vi "TestOpticalShutter.vi"() -> ()   [LabVIEW 2018]
uses:
  Mode.ctl
  Thorlabs_SC10.lvlib
panel:
  in  "stop":bool
  out "Toggle Shutter":bool
  in  "Mode":T1
  out "error out":errorcluster
  out "Connected?":bool
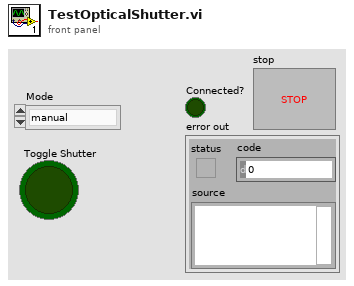
[diagram p1: front panel]
types:
  T1 = typedef "Thorlabs_SC10.lvlib/Mode.ctl" = enum16{"manual", "auto", "single", "repeat", "external gate"}
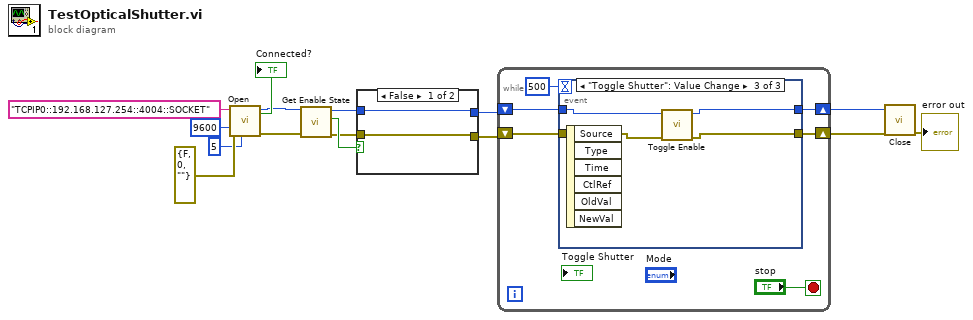
[diagram p0: block diagram]
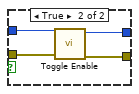
[diagram p2: hidden frame]
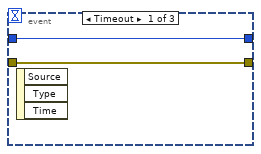
[diagram p3: hidden frame]
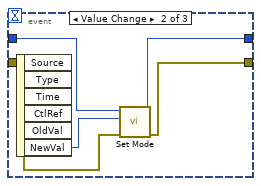
[diagram p4: hidden frame]
diagram:
  n1 = call "Open.vi"("timeout"=5, "error in (no error)"=errorcluster {"status"=FALSE, "code"=0, "source"=""}, "nbaud"=9600, "Serial Port"="TCPIP0::192.168.127.254::4004::SOCKET") -> ("error out"=w7:errorcluster, "hDevice"=w6:i32, "Connected?"=→"Connected?":bool)  [unwired: 5 in]
  n2 = call "Get Enable State.vi"("error in (no error)"=w7, "hdl"=w6) -> ("error out"=w4:errorcluster, "Enable"=w5:bool, "hdl out"=w3:i32)  [unwired: 7 in]
  n3 = case shown="False" w5 {
    tunnel: w4 -> [w16 w21]
    tunnel: w3 -> [w17 w20]
    tunnel: [w17 w19] -> w2
    tunnel: [w16 w18] -> w1
    frame False {
    }
    frame True {
      n4 = call "Toggle Enable.vi"("error in (no error)"=w21, "hdl"=w20) -> ("error out"=w18:errorcluster, "hdl out"=w19:i32)  [unwired: 8 in]
    }
  }
  n5 = while {
    shift-right: [w25] -> w9
    shift-left: w1 -> [w26]
    shift-right: [w23] -> w10
    shift-left: w2 -> [w24]
    stop <- "stop" stop-if-true
    n6 = event shown="[2] \"Toggle Shutter\": Value Change" {
      selector: _ -> [_ _ _]
      dyn-events: _ -> [_ _ _]
      timeout: 500 -> [_ _ _]
      tunnel: w26 -> [w29 w32 w37]
      tunnel: [w29 w31 w36] -> w25
      tunnel: w24 -> [w28 w33 w38]
      tunnel: [w28 w30 w35] -> w23
      event Timeout {
        n7 = event-data() -> ()  [unwired: 1 in, 3 out]
      }
      event Value Change {
        n8 = event-data() -> ("NewVal"=w34:T1)  [unwired: 1 in, 5 out]
        n9 = call "Set Mode.vi"("error in (no error)"=w32, "Mode"=w34, "hdl"=w33) -> ("error out"=w31:errorcluster, "hdl out"=w30:i32)  [unwired: 7 in]
      }
      event "Toggle Shutter": Value Change {
        n10 = event-data() -> ()  [unwired: 1 in, 6 out]
        n11 = call "Toggle Enable.vi"("error in (no error)"=w37, "hdl"=w38) -> ("error out"=w36:errorcluster, "hdl out"=w35:i32)  [unwired: 8 in]
      }
    }
  }
  n12 = call "Close.vi"("error in (no error)"=w9, "hDevice"=w10) -> ("error out"=→"error out":errorcluster)  [unwired: 9 in]
